vi "TDMS_readWave.vi"() -> ()   [LabVIEW 2011]
panel:
  out "Sine and Sawtooth":waveform(dbl)[](graph)
  out "Sines":waveform(dbl)[](graph)
  out "error out":errorcluster
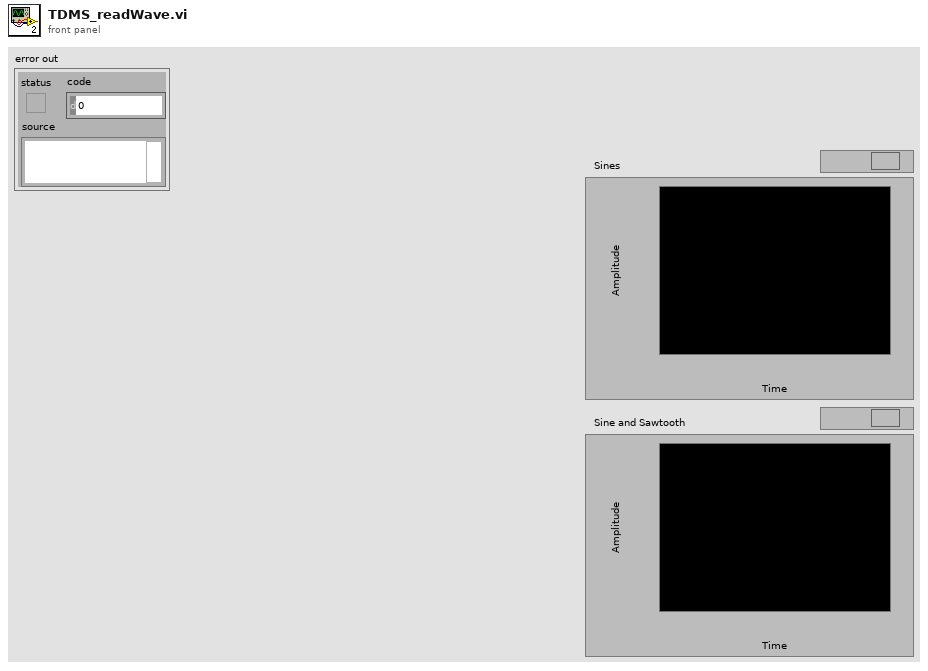
[diagram p1: front panel]
types:
  T1 = enum16{"open", "open or create", "create or replace", "create", "open (read-only)"}
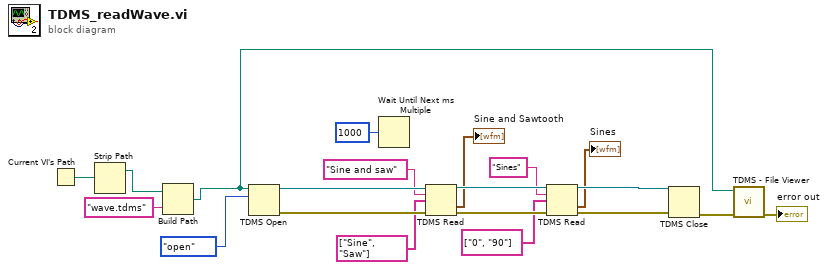
[diagram p0: block diagram]
diagram:
  n1 = Current VI's Path() -> (path=w20:path)
  n2 = Strip Path(path=w20) -> (stripped path=w19:path)  [unwired: 1 out]
  n3 = Build Path(base path=w19, name or relative path="wave.tdms") -> (appended path=w12:path)
  n4 = TDMS Open(10:T1."open" ("operation (0:open)"), 11:w12) -> (0:w15:errorcluster, 3:w16:refnum<k34>)  [unwired: 4 in]
  n5 = Wait Until Next ms Multiple(millisecond multiple=u32 1000) -> ()  [unwired: 1 out]
  n6 = TDMS Read(0:w16, 5:"Sine and saw" ("group name in (Untitled)"), 7:string[] ["Sine", "Saw"] ("channel name(s) in (Untitled)"), 11:w15) -> (4:w9:refnum<k34>, 10:→"Sine and Sawtooth":waveform(dbl)[], 15:w7:errorcluster)  [unwired: 4 in, 3 out]
  n7 = TDMS Read(0:w9, 5:"Sines" ("group name in (Untitled)"), 7:string[] ["0", "90"] ("channel name(s) in (Untitled)"), 11:w7) -> (4:w13:refnum<k34>, 10:→"Sines":waveform(dbl)[], 15:w14:errorcluster)  [unwired: 4 in, 3 out]
  n8 = TDMS Close(8:w14, 11:w13) -> (0:w11:errorcluster)  [unwired: 1 out]
  n9 = call <vilib>:"TDMS - File Viewer.vi"("error in (no error)"=w11, "file path"=w12) -> ("error out"=→"error out":errorcluster)  [unwired: 4 in, 1 out]
